vi "TCP-transmitter.vi"() -> ()   [LabVIEW 2020]
uses:
  <vilib>/numeric/Random Number (Range) I64.vi
  <vilib>/numeric/sub_Random U32.vi
panel:
  in  "stop":bool
  out "Sent data":string
  out "Num of bites":dbl
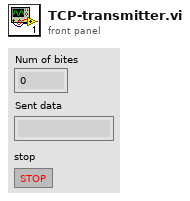
[diagram p1: front panel]
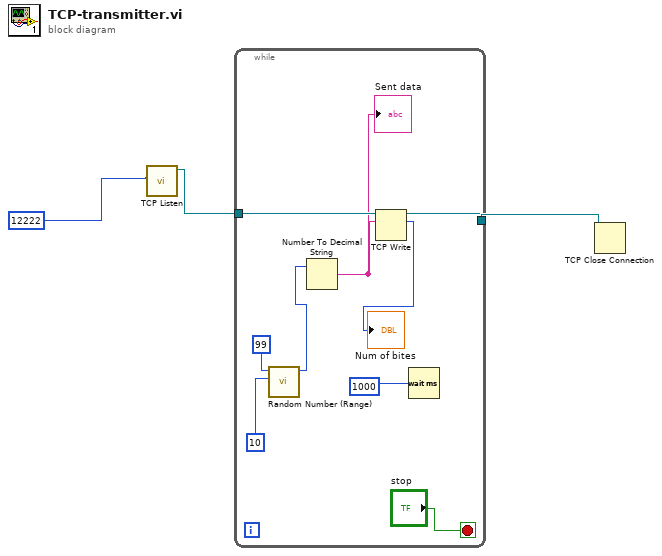
[diagram p0: block diagram]
diagram:
  n1 = call <vilib>:"TCP Listen.vi"("port"=12222) -> ("connection ID"=w1:refnum<k5>)  [unwired: 6 in, 4 out]
  n2 = while {
    tunnel: w1 -> [w12]
    tunnel: [w11] -> w3
    stop <- "stop" stop-if-true
    n3 = call-poly <vilib>:"Random Number (Range).vi"("lower bound (-100)"=10, "upper bound (100)"=99) -> ("number"=w6:i64)  [unwired: 9 in]
    n4 = Number To Decimal String(number=w6) -> (decimal integer string=w10:string)  [unwired: 1 in]
    "Sent data" <- w10
    n5 = TCP Write(connection ID=w12, data in=w10) -> (connection ID out=w11:refnum<k5>, bytes written=→"Num of bites":i32)  [unwired: 2 in, 1 out]
    n6 = Wait (ms)(milliseconds to wait=1000) -> ()  [unwired: 1 out]
  }
  n7 = TCP Close Connection(connection ID=w3) -> ()  [unwired: 2 in, 2 out]
